vi "VdRs232_Create.vi"(0 "reference":refnum<class "VdRs232.lvclass">, 1 "PortSetting (Use this settings to have full control otherwise the standalone PoartNumber and BaudeRate could be used if the DataBits=8, Parity=None and FlowControl=None)":T2={"portNbr"=enum."Com1", "baudRate"=enum."19200", "flowControl"=enum."None", "parity"=enum."None", "dataBits"=8, "stop bits (10: 1 bit)"=10} {"stop bits (10: 1 bit)" items=["1.0"=10, "1.5"=15, "2.0"=20]}, 2 "PortNumber(Ignored If Not Wired)\nThis could be a string, Enum or Int\nE.g. \"Com1\", \"2\"":variant, 3 "BaudRate(Ignored If Not Wired,19200)":T1=enum."19200", 5 "error in (no error)":errorcluster, 7 "Synchronous Mode (false)":bool, 8 "ObjectName":string) -> (14 "reference out":refnum<class "VdRs232.lvclass">, 15 "NewObjectCreated":bool=TRUE, 19 "error out":errorcluster)   [LabVIEW 2020, in "VdRs232.lvclass"]
doc: "Creates and initializes a new VdRs232 object.\n\nThis object should be destroyed using a VdRs232 destructor VI.\n\n[GOOP 2.0.13]"
uses:
  VdRs232.lvclass
  VdRs232I_ComPortType.ctl
  <vilib>/Instr/_visa.llb/VISA Find Search Mode.ctl
  <vilib>/Instr/_visa.llb/VISA Configure Serial Port (Instr).vi
  VdBaudRateType.ctl
  VdFlowControlType.ctl
  VdParityType.ctl
  ComParamsType.ctl
panel:
  # "The input reference should only\nbe wired when this method is called\nby a sub class constructor."
  # "Configure option 1"
  # "Configure option 2"
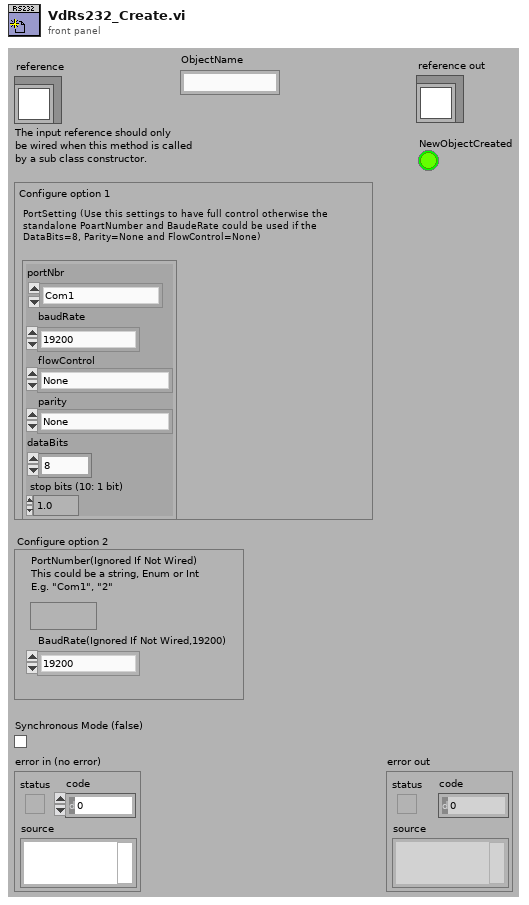
[diagram p1: front panel]
types:
  T1 = typedef "VdRs232.lvclass/VdBaudRateType.ctl" = enum16{"1200", "2400", "9600", "14400", "19200", "28800", "38400", "57600", "115200", "230400", "460800", "691200", "921600"}
  T2 = typedef "VdRs232.lvclass/ComParamsType.ctl" = cluster{"portNbr":T3, "baudRate":T1, "flowControl":T4, "parity":T5, "dataBits":u16, "stop bits (10: 1 bit)":u16}
  T3 = typedef "VdRs232.lvclass/VdRs232I_ComPortType.ctl" = enum16{"Com1", "Com2", "Com3", "Com4", "Com5", "Com6", "Com7", "Com8", "Com9", "Com10", "Com11", "Com12", "Com13", "Com14", "Com15", "Com16", "Com17", "Com18", "Com19", "Com20", "Com21", "Com22", "Com23", "Com24", "Com25", "Com26", "Com27", "Com28", "Com29", "Com30", "Com31", "Com32", "Com33", "Com34", "Com35", "Com36", "Com37", "Com38", "Com39", "Com40", "Com41", "Com42", "Com43", "Com44", "Com45", "Com46", "Com47", "Com48", "Com49", "Com50", "Com51", "Com52", "Com53", "Com54", "Com55", "Com56", "Com57", "Com58", "Com59", "Com60", "Com61", "Com62", "Com63", "Com64", "Com65", "Com66", "Com67", "Com68", "Com69", "Com70", "Com71", "Com72", "Com73", "Com74", "Com75", "Com76", "Com77", "Com78", "Com79", "Com80", "Com81", "Com82", "Com83", "Com84", "Com85", "Com86", "Com87", "Com88", "Com89", "Com90", "Com91", "Com92", "Com93", "Com94", "Com95", "Com96", "Com97", "Com98", "Com99", "Com100", "Com101", "Com102", "Com103", "Com104", "Com105", "Com106", "Com107", "Com108", "Com109", "Com110", "Com111", "Com112", "Com113", "Com114", "Com115", "Com116", "Com117", "Com118", "Com119", "Com120", "Com121", "Com122", "Com123", "Com124", "Com125", "Com126", "Com127", "Com128", "Com129", "Com130", "Com131", "Com132", "Com133", "Com134", "Com135", "Com136", "Com137", "Com138", "Com139", "Com140", "Com141", "Com142", "Com143", "Com144", "Com145", "Com146", "Com147", "Com148", "Com149", "Com150", "Com151", "Com152", "Com153", "Com154", "Com155", "Com156", "Com157", "Com158", "Com159", "Com160", "Com161", "Com162", "Com163", "Com164", "Com165", "Com166", "Com167", "Com168", "Com169", "Com170", "Com171", "Com172", "Com173", "Com174", "Com175", "Com176", "Com177", "Com178", "Com179", "Com180", "Com181", "Com182", "Com183", "Com184", "Com185", "Com186", "Com187", "Com188", "Com189", "Com190", "Com191", "Com192", "Com193", "Com194", "Com195", "Com196", "Com197", "Com198", "Com199", "Com200", "Com201", "Com202", "Com203", "Com204", "Com205", "Com206", "Com207", "Com208", "Com209", "Com210", "Com211", "Com212", "Com213", "Com214", "Com215", "Com216", "Com217", "Com218", "Com219", "Com220", "Com221", "Com222", "Com223", "Com224", "Com225", "Com226", "Com227", "Com228", "Com229", "Com230", "Com231", "Com232", "Com233", "Com234", "Com235", "Com236", "Com237", "Com238", "Com239", "Com240", "Com241", "Com242", "Com243", "Com244", "Com245", "Com246", "Com247", "Com248", "Com249", "Com250", "Com251", "Com252", "Com253", "Com254", "Com255"}
  T4 = typedef "VdRs232.lvclass/VdFlowControlType.ctl" = enum16{"None", "CTS/RTS", "XOn/XOff"}
  T5 = typedef "VdRs232.lvclass/VdParityType.ctl" = enum16{"None", "Odd", "Even"}
  T6 = enum16{"Create or look up existing", "Look up existing"}
  T7 = typedef "VdRs232.lvclass/ObjectAttributes.ctl" = cluster{"visaRef":refnum<visa-resource-name>, "portSetting":T2, "TimeoutTime(ms)":u32, "TerminationCharUsed":bool, "MatchPatternToIndicateCompleteResponse":string, "Creators":i32, "EndCharToSendForEveryMessage":string, "DefaultReadDataSize":u32, "SynchronousMode":bool, "Lock":T8}
  T8 = typedef "Semaphore RefNum" = refnum<k1>
  T9 = typedef "VISA Find Search Mode.ctl" = u32
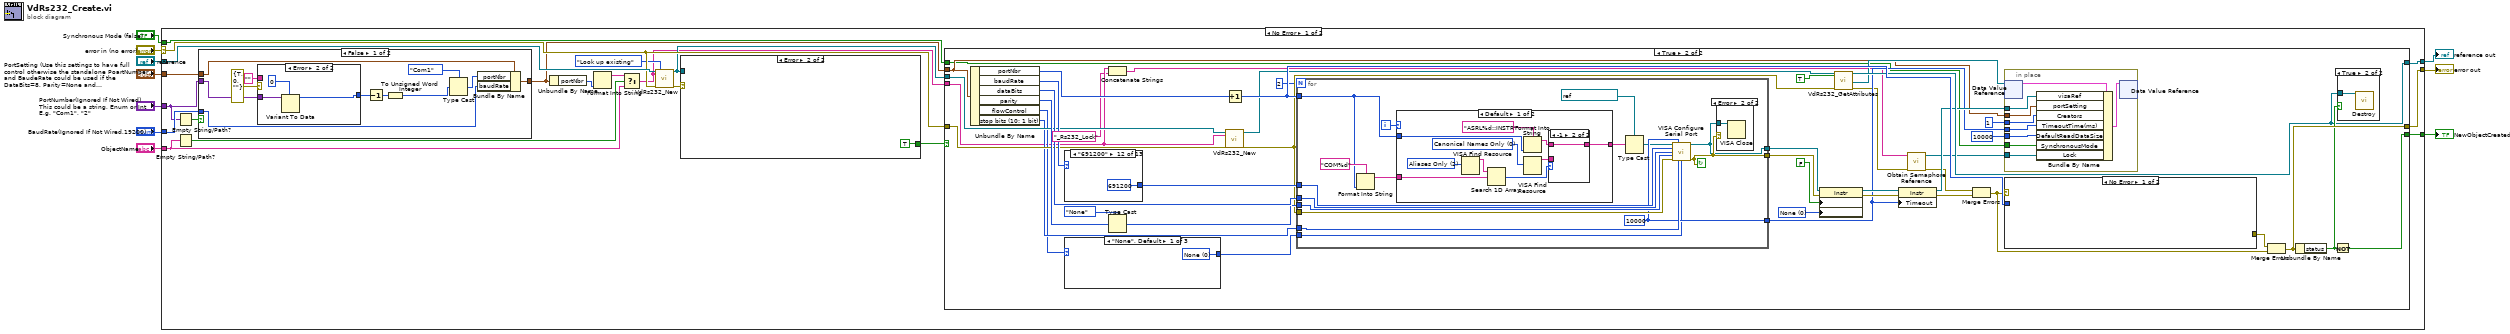
[diagram p0: block diagram]
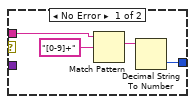
[diagram p2: hidden frame]
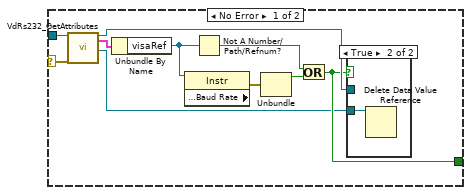
[diagram p4: hidden frame]
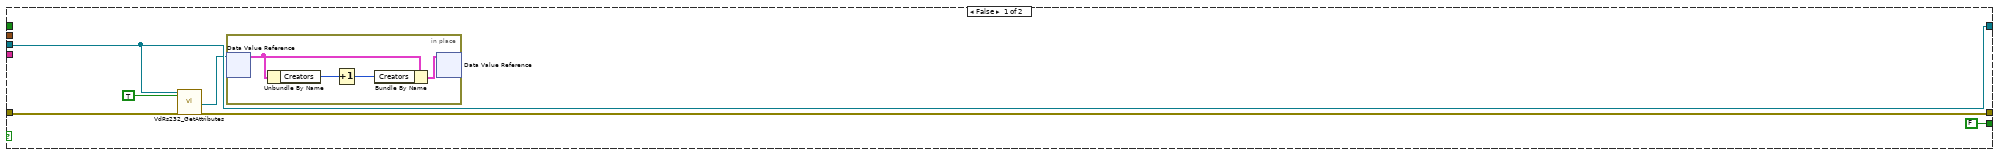
[diagram p6: hidden frame]
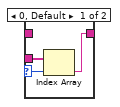
[diagram p7: hidden frame]
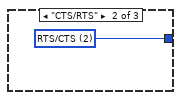
[diagram p10: hidden frame]
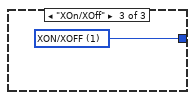
[diagram p11: hidden frame]
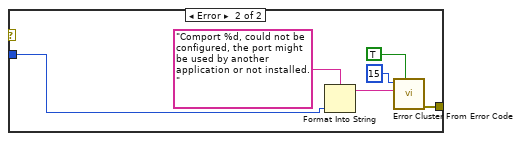
[diagram p12: hidden frame]
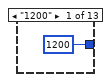
[diagram p14: hidden frame]
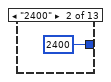
[diagram p15: hidden frame]
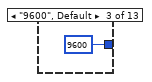
[diagram p16: hidden frame]
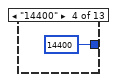
[diagram p17: hidden frame]
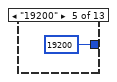
[diagram p18: hidden frame]
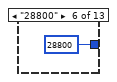
[diagram p19: hidden frame]
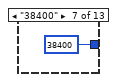
[diagram p20: hidden frame]
diagram:
  n1 = case shown="No Error" "error in (no error)" {
    selector: "error in (no error)" -> [w27 w180]
    tunnel: [w30 w179] -> w10
    tunnel: [w29 w180] -> w9
    tunnel: "reference" -> [w28 w179]
    tunnel: "PortSetting (Use this settings to have full control otherwise the standalone PoartNumber and BaudeRate could be used if the DataBits=8, Parity=None and FlowControl=None)" -> [w16 _]
    tunnel: "ObjectName" -> [w19 _]
    tunnel: [w26 _] -> w4
    tunnel: "PortNumber(Ignored If Not Wired)\nThis could be a string, Enum or Int\nE.g. \"Com1\", \"2\"" -> [w12 _]
    tunnel: "BaudRate(Ignored If Not Wired,19200)" -> [w13 _]
    tunnel: "Synchronous Mode (false)" -> [w11 _]
    frame No Error {
      n2 = Empty String/Path?(string/path=w12) -> (empty?=w14:bool)
      n3 = Empty String/Path?(string/path=w19) -> (empty?=w21:bool)
      n4 = case shown="False" w14 {
        tunnel: w16 -> [w41 w49]
        tunnel: [w40 w49] -> w15
        tunnel: w13 -> [w39 _]
        tunnel: w12 -> [w33 _]
        frame False {
          n5 = case shown="Error" errorcluster {"status"=TRUE, "code"=0, "source"=""} ("error IO") {
            tunnel: [w43 w46] -> w35
            tunnel: w33 -> [_ w47]
            tunnel: "" ("EnumValueOut(string)") -> [w42 _]
            frame No Error {
              n6 = Match Pattern(string=w42, regular expression="[0-9]+") -> (match substring=w44:string)  [unwired: 4 out]
              n7 = Decimal String To Number(string=w44) -> (number=w43:i32)  [unwired: 3 out]
            }
            frame Error {
              n8 = Variant To Data(type=0, Variant=w47) -> (data=w46:i32)  [unwired: 1 in, 1 out]
            }
          }
          n9 = Decrement(x=w35) -> (x-1=w38:i32)
          n10 = To Unsigned Word Integer(number=w38) -> (unsigned 16bit integer=w37:u16)
          n11 = Type Cast(type=VdRs232I_ComPortType."Com1" ("portNbr"), x=w37) -> (*(type *) &x=w34:T3)
          n12 = Bundle By Name(cluster=w41, "portNbr"=w34, "baudRate"=w39) -> (w40:T2)
        }
        frame True {
        }
      }
      n13 = Unbundle By Name(w15) -> ("portNbr"=w20:T3)
      n14 = Format Into String(w20) -> (resulting string=w17:string)  [unwired: 3 in, 1 out]
      n15 = Select(t=w17, s=w21, f=w19) -> (s? t:f=w18:string)
      n16 = call "VdRs232_New.vi"("reference in"=w28, "Object name"=w18, "error in (no error)"=w27, "CreateMethod(Create or look up existing)"=T6."Look up existing" ("Create method")) -> ("reference out"=w23:refnum<class "VdRs232.lvclass">, "error out"=w25:errorcluster)  [unwired: 1 in, 13 out]
      n17 = case shown="Error" w25 {
        selector: w25 -> [w58 _]
        tunnel: w23 -> [w59 _]
        tunnel: [w54 TRUE] -> w24
        frame No Error {
          n18 = call "VdRs232_GetAttributes.vi"("reference in"=w59, "error in (no error)"=w58) -> ("reference out"=w57:refnum<class "VdRs232.lvclass">, "Data"=w51:T7, "DataRef"=w50:refnum<data-value>)  [unwired: 1 in, 14 out]
          n19 = Unbundle By Name(w51) -> ("visaRef"=w56:refnum<visa-resource-name>)
          n20 = property class="Instr" props=["Serial Settings:Baud Rate"](reference=w56) -> (error out=w55:errorcluster)  [unwired: 1 in, 2 out]
          n21 = Not A Number/Path/Refnum?(number/path/refnum=w56) -> (NaN/Path/Refnum?=w53:bool)
          n22 = Unbundle(w55) -> ("status"=w52:bool)  [unwired: 2 out]
          n23 = Or(x=w53, y=w52) -> (x .or. y?=w54:bool)
          n24 = case shown="True" w54 {
            tunnel: w57 -> [_ _]
            tunnel: w50 -> [_ w60]
            frame False {
            }
            frame True {
              n25 = Delete Data Value Reference(data value reference=w60) -> ()  [unwired: 1 in, 2 out]
            }
          }
        }
        frame Error {
        }
      }
      n26 = case shown="True" w24 {
        tunnel: [w65 w97] -> w30
        tunnel: [w64 w100] -> w29
        tunnel: w15 -> [_ w83]
        tunnel: w27 -> [w66 w101]
        tunnel: [FALSE w99] -> w26
        tunnel: w18 -> [_ w75]
        tunnel: w23 -> [w65 w93]
        tunnel: w11 -> [_ w79]
        frame False {
          n27 = call "VdRs232_GetAttributes.vi"("reference in"=w65, "OnlyGetDvrReference(False)"=TRUE, "error in (no error)"=w66) -> ("DataRef"=w62:refnum<data-value>, "error out"=w64:errorcluster)  [unwired: 13 in, 2 out]
          n28 = in-place {
            n29 = in-place-dvr #1(w62) -> (w71:T7)  [unwired: 1 out]
            n30 = Unbundle By Name(w71) -> ("Creators"=w70:i32)
            n31 = Increment(x=w70) -> (x+1=w69:i32)
            n32 = Bundle By Name(cluster=w71, "Creators"=w69) -> (w68:T7)
            n33 = in-place-dvr #1(w68) -> ()  [unwired: 2 out]
          }
        }
        frame True {
          w102 = u16 0 items=["None", "Last Bit", "TermChar"] ("Serial Settings:Serial End Mode for Reads")
          n34 = Unbundle By Name(w83) -> ("portNbr"=w114:T3, "baudRate"=w109:T1, "dataBits"=w113:u16, "parity"=w112:T5, "flowControl"=w88:T4, "stop bits (10: 1 bit)"=w92:u16)
          n35 = case shown="\"691200\"" w109 {
            tunnel: [u32 1200 ("baud rate (9600)") u32 2400 ("baud rate (9600)") u32 9600 ("baud rate (9600)") u32 14400 ("baud rate (9600)") u32 19200 ("baud rate (9600)") u32 28800 ("baud rate (9600)") u32 38400 ("baud rate (9600)") u32 57600 ("baud rate (9600)") u32 115200 ("baud rate (9600)") u32 230400 ("baud rate (9600)") u32 460800 ("baud rate (9600)") u32 691200 ("baud rate (9600)") u32 921600 ("baud rate (9600)")] -> w108
            frame "1200" {
            }
            frame "2400" {
            }
            frame "9600", Default {
            }
            frame "14400" {
            }
            frame "19200" {
            }
            frame "28800" {
            }
            frame "38400" {
            }
            frame "57600" {
            }
            frame "115200" {
            }
            frame "230400" {
            }
            frame "460800" {
            }
            frame "691200" {
            }
            frame "921600" {
            }
          }
          n36 = case shown="\"None\", Default" w88 {
            tunnel: [w156 w157 w158] -> w87
            frame "None", Default {
              w156 = u16 0 items=["None", "XON/XOFF", "RTS/CTS", "XON/XOFF & RTS/CTS", "DTR/DSR", "XON/XOFF & DTR/DSR"] ("flow control (0:none)")
            }
            frame "CTS/RTS" {
              w157 = u16 2 items=["None", "XON/XOFF", "RTS/CTS", "XON/XOFF & RTS/CTS", "DTR/DSR", "XON/XOFF & DTR/DSR"] ("flow control (0:none)")
            }
            frame "XOn/XOff" {
              w158 = u16 1 items=["None", "XON/XOFF", "RTS/CTS", "XON/XOFF & RTS/CTS", "DTR/DSR", "XON/XOFF & DTR/DSR"] ("flow control (0:none)")
            }
          }
          n37 = Concatenate Strings(w75, "_Rs232_Lock" ("string")) -> (w74:string)
          n38 = Type Cast(type=enum16{"None", "Odd", "Even", "Mark", "Space"}."None" ("parity (0:none)"), x=w112) -> (*(type *) &x=w111:enum16{"None", "Odd", "Even", "Mark", "Space"})
          n39 = call "VdRs232_New.vi"("reference in"=w93, "Object name"=w75, "error in (no error)"=w101) -> ("reference out"=w96:refnum<class "VdRs232.lvclass">, "error out"=w95:errorcluster)  [unwired: 1 in, 14 out]
          n40 = Increment(x=w114) -> (x+1=w106:T3)
          n41 = for {
            N: 2 -> [_]
            tunnel: w113 -> [w139]
            tunnel: w111 -> [w138]
            tunnel: w108 -> [w137]
            tunnel: w106 -> [w124]
            tunnel: [w131] -> w105
            tunnel: [w132] -> w103
            tunnel: w95 -> [w136]
            tunnel: w92 -> [w135]
            tunnel: [w134] -> w81
            tunnel: w87 -> [w133]
            i -> [w130]
            stop <- w132 continue-if-true
            w134 = u32 10000 ("timeout (10sec)")
            n42 = Format Into String(format string="COM%d" ("Format String"), w124) -> (resulting string=w127:string)  [unwired: 2 in, 1 out]
            n43 = case shown="Default" w130 {
              tunnel: [w143 w154] -> w126
              tunnel: w127 -> [w146 w154]
              tunnel: w124 -> [w141 _]
              frame Default {
                w148 = T9 0 items=["Canonical Names Only"=0, "Aliases Only"=2, "Include Matching Aliases"=3, "Include All Aliases"=4] ("Search Mode")
                w149 = T9 2 items=["Canonical Names Only"=0, "Aliases Only"=2, "Include Matching Aliases"=3, "Include All Aliases"=4] ("Search Mode")
                n44 = VISA Find Resource(10:w149) -> (3:w147:string[])  [unwired: 2 in, 2 out]
                n45 = Search 1D Array(1D array=w147, element=w146) -> (index of element=w145:i32)  [unwired: 1 in]
                n46 = Format Into String(format string="ASRL%d::INSTR" ("Format String"), w141) -> (resulting string=w140:string)  [unwired: 2 in, 1 out]
                n47 = VISA Find Resource(10:w148) -> (3:w144:string[])  [unwired: 2 in, 2 out]
                n48 = case shown="-1" w145 {
                  selector: w145 -> [w152 _]
                  tunnel: w144 -> [w151 _]
                  tunnel: [w150 w153] -> w143
                  tunnel: w140 -> [_ w153]
                  frame 0, Default {
                    n49 = Index Array(array=w151, index=w152) -> (element=w150:string)
                  }
                  frame -1 {
                  }
                }
              }
              frame 0 {
              }
            }
            n50 = Type Cast(type=refnum<visa-resource-name> "ASRL2::INSTR" ("VISA resource name"), x=w126) -> (*(type *) &x=w128:refnum<visa-resource-name>)
            n51 = call-poly "VISA Configure Serial Port"("VISA resource name"=w128, "timeout (10sec)"=w134, "baud rate (9600)"=w137, "data bits (8)"=w139, "parity (0:none)"=w138, "error in (no error)"=w136, "stop bits (10: 1 bit)"=w135, "flow control (0:none)"=w133) -> ("VISA resource name out"=w131:refnum<visa-resource-name>, "error out"=w132:errorcluster)  [unwired: 6 out]
            n52 = case shown="Error" w132 {
              tunnel: w131 -> [_ w155]
              frame No Error {
              }
              frame Error {
                n53 = VISA Close(VISA resource name=w155) -> ()  [unwired: 1 in, 1 out]
              }
            }
          }
          n54 = property class="Instr"(reference=w105, error in=w103, "Message Based Settings:Termination Character Enable"=FALSE, "Serial Settings:End Mode for Reads"=w102) -> (reference out=w89:refnum<visa-resource-name>, error out=w91:errorcluster)
          n55 = call "VdRs232_GetAttributes.vi"("reference in"=w96, "OnlyGetDvrReference(False)"=TRUE, "error in (no error)"=w95) -> ("reference out"=w97:refnum<class "VdRs232.lvclass">, "DataRef"=w85:refnum<data-value>, "error out"=w78:errorcluster)  [unwired: 13 in, 1 out]
          n56 = property class="Instr"(reference=w89, error in=w91, "Timeout"=w81) -> (reference out=w84:refnum<visa-resource-name>, error out=w90:errorcluster)
          n57 = call <vilib>:"Obtain Semaphore Reference.vi"("error in (no error)"=w78, "name (unnamed)"=w74) -> ("error out"=w77:errorcluster, "semaphore"=w76:T8)  [unwired: 3 in, 1 out]
          n58 = Merge Errors(w77, w90) -> (w94:errorcluster)
          n59 = in-place {
            in-place-border: w84 -> [w122]
            in-place-border: w83 -> [w121]
            in-place-border: 1 ("Creators") -> [w120]
            in-place-border: w81 -> [w119]
            in-place-border: u32 10000 ("DefaultReadDataSize") -> [w118]
            in-place-border: w79 -> [w117]
            in-place-border: w76 -> [w115]
            n60 = in-place-dvr #2(w85) -> (w123:T7)  [unwired: 1 out]
            n61 = Bundle By Name(cluster=w123, "visaRef"=w122, "portSetting"=w121, "Creators"=w120, "TimeoutTime(ms)"=w119, "DefaultReadDataSize"=w118, "SynchronousMode"=w117, "Lock"=w115) -> (w116:T7)
            n62 = in-place-dvr #2(w116) -> ()  [unwired: 2 out]
          }
          n63 = case shown="No Error" w94 {
            tunnel: [_ w161] -> w107
            tunnel: w106 -> [_ w160]
            frame No Error {
            }
            frame Error {
              n64 = Format Into String(format string="Comport %d, could not be configured, the port might be used by another application or not installed." ("source"), w160) -> (resulting string=w162:string)  [unwired: 2 in, 1 out]
              n65 = call <vilib>:"Error Cluster From Error Code.vi"("show call chain? (False)"=TRUE, "error message (\"\")"=w162, "error code (0)"=15 ("code (5000)")) -> ("error out"=w161:errorcluster)  [unwired: 1 in, 5 out]
            }
          }
          n66 = Merge Errors(w107, w94) -> (w100:errorcluster)
          n67 = Unbundle By Name(w100) -> ("status"=w98:bool)
          n68 = Not(x=w98) -> (.not. x?=w99:bool)
          n69 = case shown="True" w98 {
            tunnel: w97 -> [_ w165]
            frame False {
            }
            frame True {
              n70 = call "Destroy.vi"("reference"=w165) -> ()  [unwired: 1 in, 18 out]
            }
          }
        }
      }
    }
    frame Error {
      (unwired) -1 ("Nr of open handles")
    }
  }
  "error out" <- w9
  "reference out" <- w10
  "NewObjectCreated" <- w4
